vi "Set Init Complete.vi"(8 "error in (no error)":errorcluster, 10 "Initialization Complete":bool, 11 "FPGA VI Reference in":T1) -> (0 "error out":errorcluster, 3 "FPGA VI Reference out":T1)   [LabVIEW 2009]
uses:
  <vilib>/rvi/interface/nirviReadWriteControl/nirviReadWriteControl.xnode
  TypeDefs/Sensor TypeDefs/FPGA Main ref.ctl
  FPGA Bitfiles/Q_IGVC_2010.lvproj_FPGA Target_FPGA_MAIN.vi.lvbitx
  <vilib>/RVI Host/nirviSupport.llb/nirviErrorClusterFromErrorCode.vi
  <vilib>/rvi/errors/niLvFpgaWhatHappensToTopLevelVI.ctl
  <vilib>/rvi/interface/common/niFpgaNodeNameForErrorReporting.ctl
  <vilib>/rvi/errors/niLvFpgaAdjustHostInterfaceError.vi
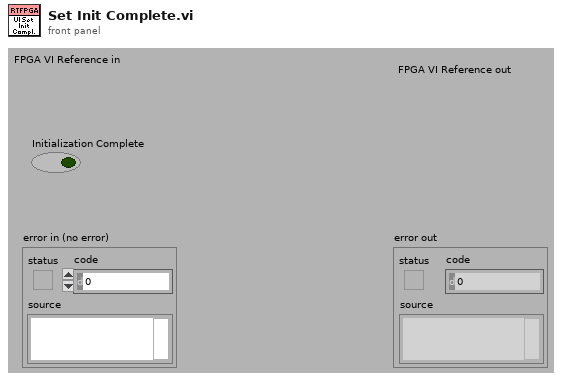
[diagram p1: front panel]
types:
  T1 = typedef "FPGA Main ref.ctl" = refnum<k20>
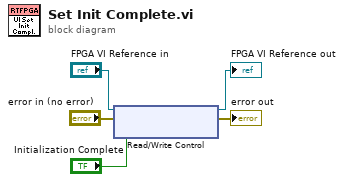
[diagram p0: block diagram]
diagram:
  n1 = xnode "Read/Write Control"("FPGA VI Reference In"="FPGA VI Reference in", "error in"="error in (no error)", "UI Init Complete"="Initialization Complete") -> ("FPGA VI Reference Out"=→"FPGA VI Reference out":T1, "error out"=→"error out":errorcluster)
